vi "Before Each.vi"(8 "Error In":errorcluster, 11 "Data":string) -> (0 "Error Out":errorcluster, 3 "Reader":refnum<class "Reader.lvclass">)   [LabVIEW 2018, in "Tests.lvlib" / "Reader.lvlib"]
uses:
  Reader.lvlib
  src/Toolkit/Public/Reader/Reader.lvclass
  src/Toolkit/Public/Reader/Private/Begin by Value.vi
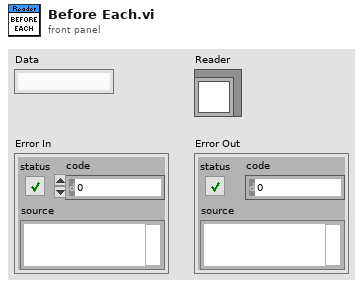
[diagram p1: front panel]
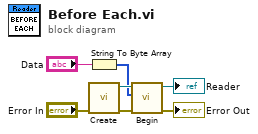
[diagram p0: block diagram]
diagram:
  n1 = String To Byte Array(string="Data") -> (unsigned byte array=w5:u8[])
  n2 = call "Create.vi"("Error In"="Error In") -> ("Error Out"=w7:errorcluster, "Reader"=w6:refnum<class "Reader.lvclass">)  [unwired: 9 in]
  n3 = call-poly "Begin.vi"("Error In"=w7, "Msgpack Data"=w5, "Reader In"=w6) -> ("Error Out"=→"Error Out":errorcluster, "Reader Out"=→"Reader":refnum<class "Reader.lvclass">)  [unwired: 7 in]
